vi "FTW-TestExecutive-Core_Step_Complete.vi"(0 "FTW-TestExecutive-Core In":refnum<class "FTW-TestExecutive-Core.lvclass">, 7 "Results":T1 {"Start Time" format="%<%Y-%m-%d %H:%M:%S%03u>T"; "Elapsed Time" format="%<%H:%M:%S%3u>t"}, 11 "error in":errorcluster) -> (4 "FTW-TestExecutive-Core Out":refnum<class "FTW-TestExecutive-Core.lvclass">, 15 "error out":errorcluster)   [LabVIEW 2015, in "FTW-TestExecutive-Core.lvclass"]
uses:
  FTW-TestExecutive-Core.lvclass
  FTW-TestExecutive-Results.ctl
  FTW-TestExecutive-Step-State.ctl
  FTW-TestExecutive-Core.lvclass/FTW-TestExecutive-Core.ctl
  FTW-TestExecutive-Core_State.ctl
  source/actor/Connector/FTW-ActorConnector.lvclass
  source/actor/Instance/FTW-ActorInstance.lvclass
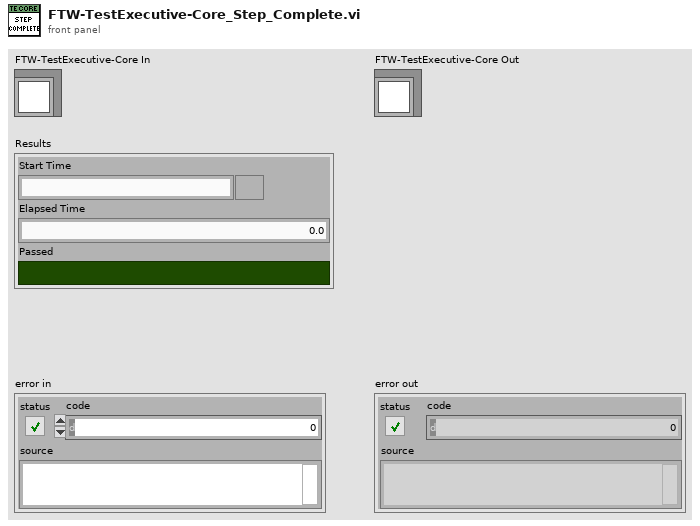
[diagram p1: front panel]
types:
  T1 = typedef "FTW-TestExecutive-Results.ctl" = cluster{"Start Time":timestamp, "Elapsed Time":dbl, "Passed":bool}
  T2 = typedef "FTW-TestExecutive-Step-State.ctl" = enum8{"None", "Failed", "Passed", "Timed out", "Aborted"}
  T3 = typedef "FTW-TestExecutive-Core.lvclass/FTW-TestExecutive-Core_State.ctl" = enum8{"Unloaded", "Loaded", "Executing", "Paused"}
  T4 = typedef "FTW-TestExecutive-Step.ctl" = cluster{"Name":string, "Type":string, "Path":string, "Config":string, "Elapsed Time":dbl, "Passed":bool, "State":T2, "Results":T1}
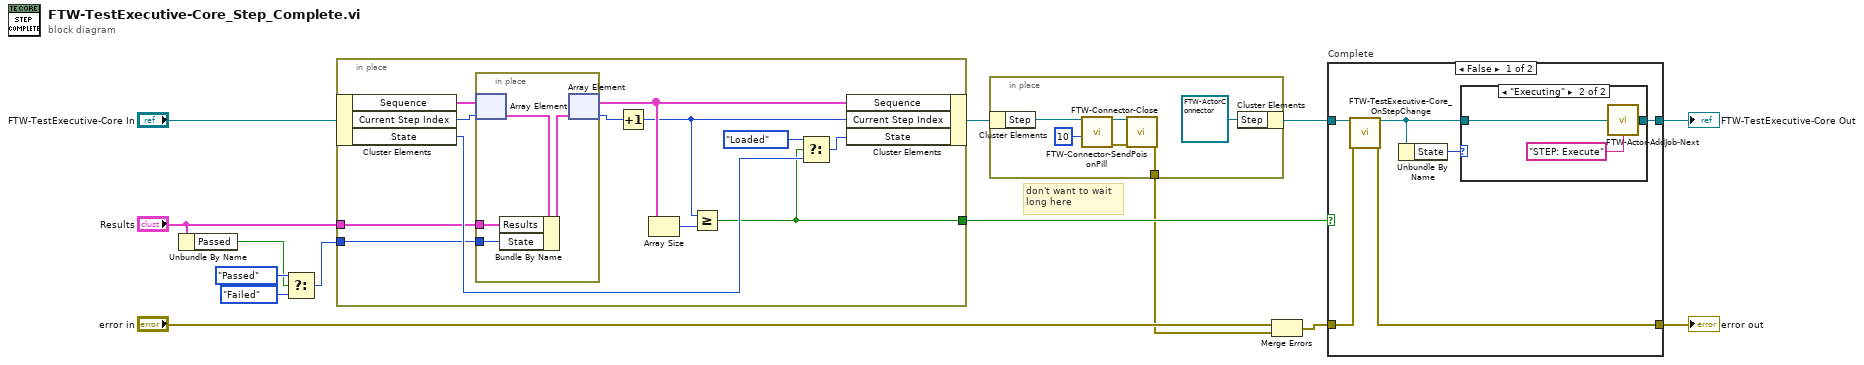
[diagram p0: block diagram]
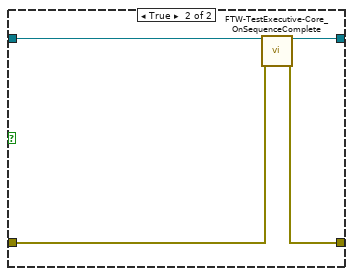
[diagram p3: hidden frame]
diagram:
  # "don't want to wait\nlong here"
  n1 = Unbundle By Name("Results") -> ("Passed"=w9:bool)
  n2 = Select(t=FTW-TestExecutive-Step-State."Passed" ("State"), s=w9, f=FTW-TestExecutive-Step-State."Failed") -> (s? t:f=w12:T2)
  n3 = in-place {
    in-place-border: "Results" -> [w23]
    in-place-border: w12 -> [w22]
    in-place-border: [w15] -> w6
    n4 = in-place-cluster #1("FTW-TestExecutive-Core In") -> ("Sequence"=w24:T4[], "Current Step Index"=w21:i32, "State"=w26:T3)
    n5 = in-place {
      in-place-border: w23 -> [w28]
      in-place-border: w22 -> [w27]
      n6 = in-place-array #2(w24, w21) -> (w30:T4)
      n7 = Bundle By Name(cluster=w30, "Results"=w28, "State"=w27) -> (w29:T4)
      n8 = in-place-array #2(w29) -> (w25:T4[], w20:i32)
    }
    n9 = Increment(x=w20) -> (x+1=w19:i32)
    n10 = Array Size(array=w25) -> (size(s)=w18:i32)
    n11 = Greater Or Equal?(x=w19, y=w18) -> (x >= y?=w15:bool)
    n12 = Select(t=FTW-TestExecutive-Core_State."Loaded" ("State"), s=w15, f=w26) -> (s? t:f=w16:T3)
    n13 = in-place-cluster #1("Sequence"=w25, "Current Step Index"=w19, "State"=w16) -> (w2:refnum<class "FTW-TestExecutive-Core.lvclass">)
  }
  n14 = in-place {
    in-place-border: [w34] -> w3
    n15 = in-place-cluster #3(w2) -> ("Step"=w32:refnum<class "FTW-ActorConnector.lvclass">)
    n16 = call-dynamic "FTW-Connector-SendPoisonPill.vi"("FTW Actor Connector"=w32, "Timeout"=10) -> ("FTW Actor Connector out"=w36:refnum<class "FTW-ActorConnector.lvclass">, "error out"=w35:errorcluster)  [unwired: 8 in, 4 out]
    n17 = call-dynamic "FTW-Connector-Close.vi"("FTW Actor Connector"=w36, "error in"=w35) -> ("error out"=w34:errorcluster)  [unwired: 13 in]
    n18 = in-place-cluster #3("Step"=refnum<class "FTW-ActorConnector.lvclass"> refnum) -> (w1:refnum<class "FTW-TestExecutive-Core.lvclass">)
  }
  n19 = Merge Errors("error in", w3) -> (w4:errorcluster)
  n20 = case "Complete" shown="False" w6 {
    tunnel: w1 -> [w42 w50]
    tunnel: [w41 w49] -> w8
    tunnel: w4 -> [w40 w48]
    tunnel: [w39 w47] -> w7
    frame False {
      n21 = call "FTW-TestExecutive-Core_OnStepChange.vi"("FTW-TestExecutive-Core In"=w42, "error in"=w40) -> ("FTW-TestExecutive-Core Out"=w38:refnum<class "FTW-TestExecutive-Core.lvclass">, "error out"=w39:errorcluster)  [unwired: 12 in]
      n22 = Unbundle By Name(w38) -> ("State"=w37:T3)
      n23 = case shown="\"Executing\"" w37 {
        tunnel: w38 -> [w43 w46]
        tunnel: [w43 w45] -> w41
        frame "Unloaded", "Loaded", "Paused" {
        }
        frame "Executing" {
          n24 = call "FTW-Actor-AddJob-Next.vi"("Add Next in Job Queue"="STEP: Execute", "FTW Actor Instance"=w46) -> ("FTW Actor Instance out"=w45:refnum<class "FTW-TestExecutive-Core.lvclass">)  [unwired: 2 in]
        }
      }
    }
    frame True {
      n25 = call "FTW-TestExecutive-Core_OnSequenceComplete.vi"("FTW-TestExecutive-Core In"=w50, "error in"=w48) -> ("FTW-TestExecutive-Core Out"=w49:refnum<class "FTW-TestExecutive-Core.lvclass">, "error out"=w47:errorcluster)  [unwired: 12 in]
    }
  }
  "FTW-TestExecutive-Core Out" <- w8
  "error out" <- w7
